vi "read-File-&-Plot-XY.vi"() -> ()   [LabVIEW 2024]
panel:
  out "filenames":string[](array[string])
  out "XY Graph":T1(graph)
  out "array":dbl[][](array[numeric])
  out "text":string
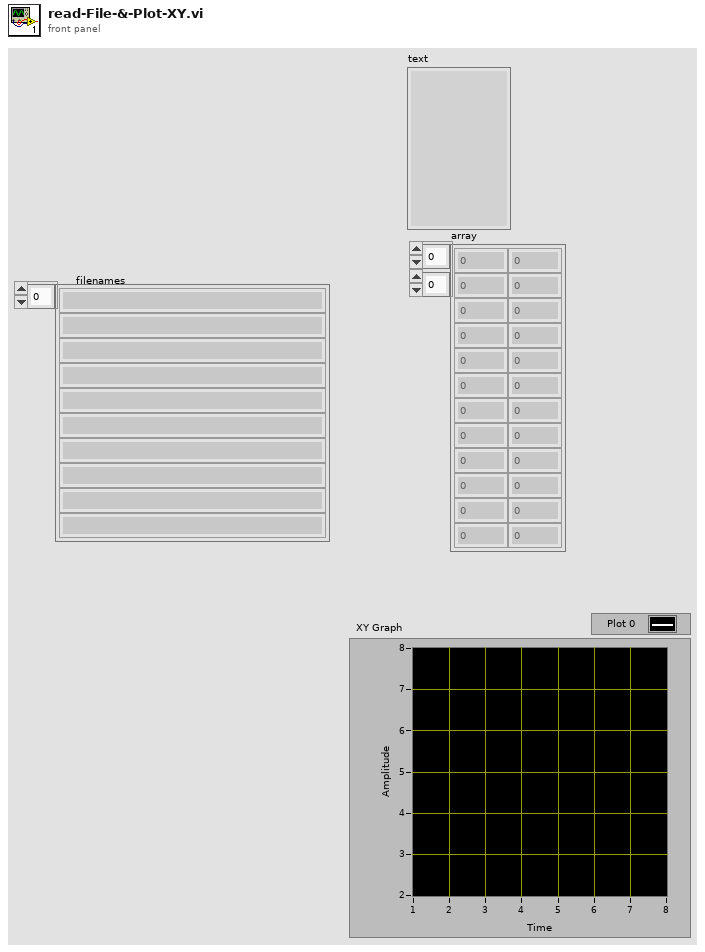
[diagram p1: front panel]
types:
  T1 = cluster{"array type (2D Dbl)":dbl[], "array type (2D Dbl)":dbl[]}
  T2 = enum16{"open", "replace", "create", "open or create", "replace or create", "replace or create with confirmation"}
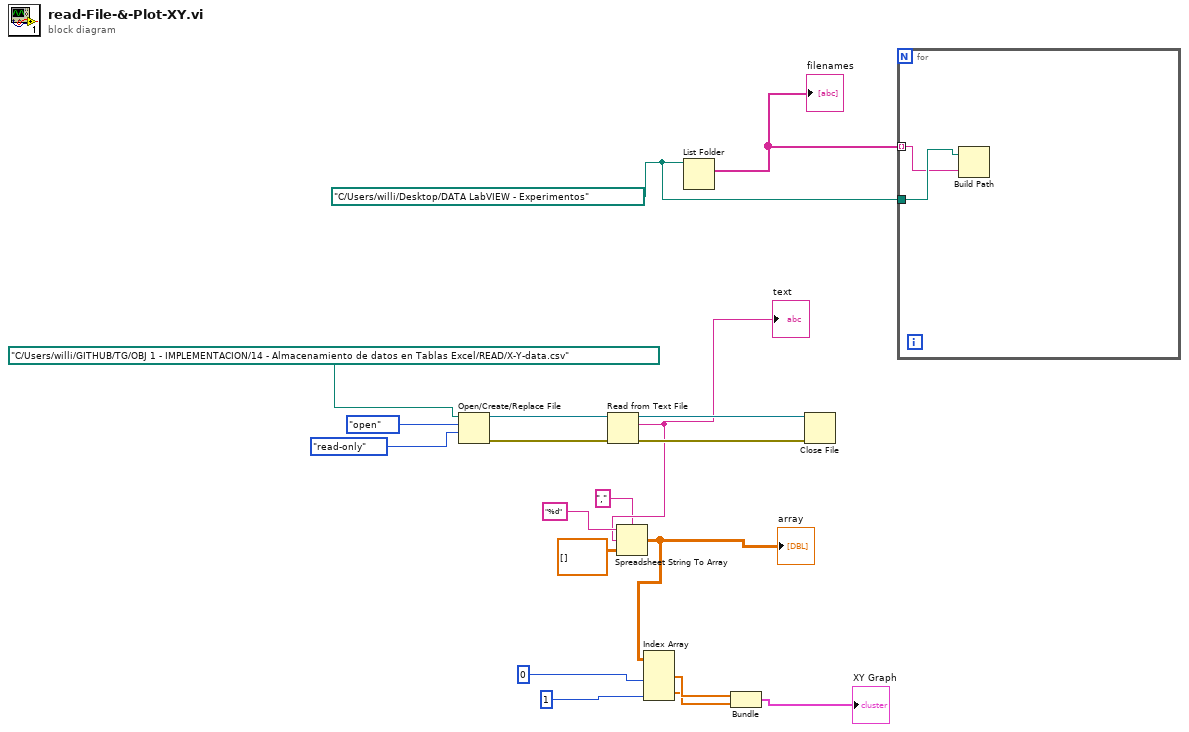
[diagram p0: block diagram]
diagram:
  w1 = path "C:/Users/willi/Desktop/DATA LabVIEW - Experimentos" ("path")
  n1 = Open/Create/Replace File(file path (use dialog)=path "C:/Users/willi/GITHUB/TG/OBJ 1 - IMPLEMENTACION/14 - Almacenamiento de datos en Tablas Excel/READ/X-Y-data.csv", operation (0:open)=T2."open", access (0:read/write)=enum16{"read/write", "read-only", "write-only"}."read-only") -> (refnum out=w19:refnum<file>, error out=w16:errorcluster)  [unwired: 3 in, 1 out]
  n2 = Read from Text File(file (use dialog)=w19, error in=w16) -> (refnum out=w18:refnum<file>, text=w12:string, error out=w15:errorcluster)  [unwired: 2 in, 1 out]
  "text" <- w12
  n3 = Spreadsheet String To Array(delimiter (Tab)=",", format string="%d", spreadsheet string=w12, array type (2D Dbl)=dbl[][] []) -> (array=w9:dbl[][])
  "array" <- w9
  n4 = Index Array(array=w9, index (col) #1=0 ("index"), index (col) #2=1 ("index")) -> (element #1=w6:dbl[], element #2=w5:dbl[])  [unwired: 2 in]
  n5 = List Folder(path=w1) -> (filenames=w2:string[])  [unwired: 3 in, 3 out]
  "filenames" <- w2
  n6 = Bundle("array type (2D Dbl)"=w6, "array type (2D Dbl)"=w5) -> (→"XY Graph":T1)  [unwired: 1 in]
  n7 = Close File(refnum=w18, error in=w15) -> ()  [unwired: 2 out]
  n8 = for {
    tunnel: w2 -> [w20] mode=indexing
    tunnel: w1 -> [w21]
    n9 = Build Path(base path=w21, name or relative path=w20) -> ()  [unwired: 1 out]
  }
